vi "Replication and Deployment Utility.vi"() -> ()   [LabVIEW 2020]
uses:
  subVIs/Util/FP Control/FP Control Functions.ctl
  subVIs/rad_Globals.vi
  subVIs/Util/Controls/Exit Button.ctl
  <vilib>/Utility/miscctls.llb/LVRowAndColumnUnsignedTypeDef.ctl
  subVIs/Util/Controls/Refresh Button.ctl
  subVIs/Util/Controls/Retrieve Button.ctl
  subVIs/Util/Controls/Configure Button.ctl
  subVIs/TypeDefs/rad_State Data.ctl
  subVIs/App Images/TypeDefs/rad_Application Image Properties.ctl
  subVIs/App Images/TypeDefs/rad_App Images Settings.ctl
  subVIs/Targets/TypeDefs/rad_Targets Settings.ctl
  subVIs/App Images/TypeDefs/rad_AppImage Information.ctl
  subVIs/Util/Controls/Deploy Button.ctl
  subVIs/Util/Controls/Select All Button.ctl
  subVIs/App Images/TypeDefs/rad_FPGA Properties.ctl
  subVIs/App Images/TypeDefs/rad_FPGA Flash Properties.ctl
  subVIs/Util/Controls/Add Target Button.ctl
  subVIs/Targets/TypeDefs/rad_Target Information.ctl
  subVIs/Targets/TypeDefs/rad_Target Network Settings.ctl
panel:
  in  "Password":string
  in  "Targets Settings":bool
  in  "Refresh Targets":T1
  in  "Target List":i32[](listbox)
  in  "Add Target":T2
  in  "Select All":T3
  in  "Configure Targets":T4
  in  "Deploy":T5
  in  "Retrieve":T6
  in  "State":T7={"Targets Settings"={"Target Types"=["cRIO"], "Reduce Discovery Timeout"=TRUE}, "Targets Information"=[], "App Images Settings"={"App Images Folder"=path "C:/work/cRIO images", "App Images Temp Folder"=path "C:/Users/admin/AppData/Local/Temp/lvtemporary_671449.rad", "CurrentVersion"=""}, "App Images Information"=[], "Filtered Targets"=[], "AppMode"="Manager", "Configuration File Path"=path "C:/work/zaphiro_gtools/Sources/Utilities/rad_16_0_source/rad_config.ini", "Permissions"={"Retrieve AppImgs"=TRUE}, "User Added Targets"=["169.254.1.19"]} {"Targets Information"."Primary NIC"."IP Address Request Mode" items=["Static"=1, "DHCP/Link-Local"=2, "Link-Local Only"=4, "DHCP Only"=8]}
  in  "App Images Settings":bool
  in  "Refresh Apps":T1
  in  "Exit":T16
  in  "App Images List":i32(listbox)=-1
  in  "Configure App":T4
  # "Deployment Targets"
  # "Application Images"
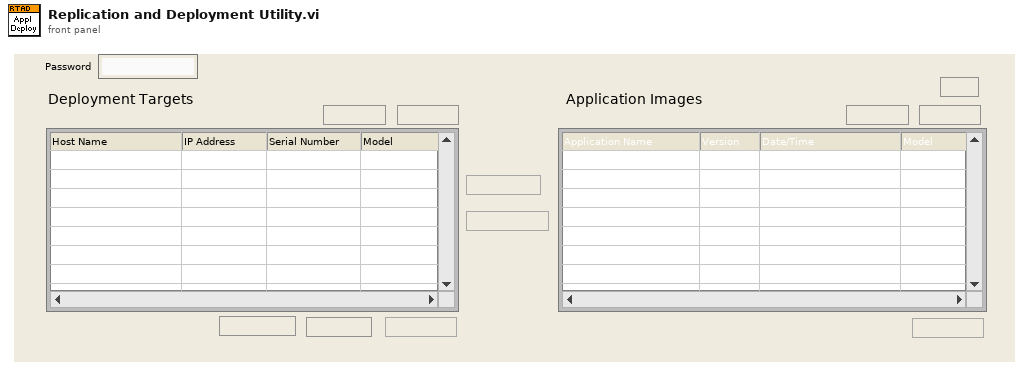
[diagram p1: front panel]
types:
  T1 = typedef "Refresh Button.ctl" = bool
  T2 = typedef "Add Target Button.ctl" = bool
  T3 = typedef "Select All Button.ctl" = bool
  T4 = typedef "Configure Button.ctl" = bool
  T5 = typedef "Deploy Button.ctl" = bool
  T6 = typedef "Retrieve Button.ctl" = bool
  T7 = typedef "rad_State Data.ctl" = cluster{"Targets Settings":T8, "Targets Information":T9[], "App Images Settings":T11, "App Images Information":T12[], "Filtered Targets":i32[], "AppMode":string, "Configuration File Path":path, "Permissions":cluster{"Retrieve AppImgs":bool}, "User Added Targets":string[]}
  T8 = typedef "rad_Targets Settings.ctl" = cluster{"Target Types":string[], "Reduce Discovery Timeout":bool}
  T9 = typedef "rad_Target Information.ctl" = cluster{"Hostname":string, "Serial number":string, "Product name":string, "Product code":i32, "System status":string, "Credential type":enum16{"None/Unlocked", "FTP Password", "NIAuth Credentials"}, "User added?":bool, "Primary NIC":T10}
  T10 = typedef "rad_Target Network Settings.ctl" = cluster{"MAC address":string, "IP Address Request Mode":i32, "IP address":string, "Subnet mask":string, "Gateway":string, "DNS server":string}
  T11 = typedef "rad_App Images Settings.ctl" = cluster{"App Images Folder":path, "App Images Temp Folder":path, "CurrentVersion":string}
  T12 = typedef "rad_AppImage Information.ctl" = cluster{"AppImage Properties":T13, "AppImage Path":path}
  T13 = typedef "rad_Application Image Properties.ctl" = cluster{"Name":string, "Version":string, "Time":timestamp, "Description":string, "Key":string, "Chassis":string, "FPGA Properties":T14, "Model":string, "Retrieve":string[], "Deploy":string[], "Installed Software":string[]}
  T14 = typedef "rad_FPGA Properties.ctl" = T15[]
  T15 = typedef "rad_FPGA Flash Properties.ctl" = cluster{"Resource Name":string, "Path":path}
  T16 = typedef "Exit Button.ctl" = bool
  T17 = typedef "LVPoint32TypeDef.ctl" = cluster{"Horizontal":i32, "Vertical":i32}
  T18 = typedef "LVRowAndColumnTypeDef.ctl" = cluster{"Row":i32, "Column":i32}
  T19 = typedef "FP Control Functions.ctl" = enum16{"Open", "Close", "Bring To Front", "Center"}
  T20 = typedef "LVRowAndColumnUnsignedTypeDef.ctl" = cluster{"Row":u32, "Column":u32}
  T21 = enum8{"Enabled", "Disabled", "Disabled and Grayed Out"}
  T22 = enum32{"invalid app kind", "Development System", "Run Time System", "Student Edition", "Embedded LabVIEW", "Evaluation", "Custom"}
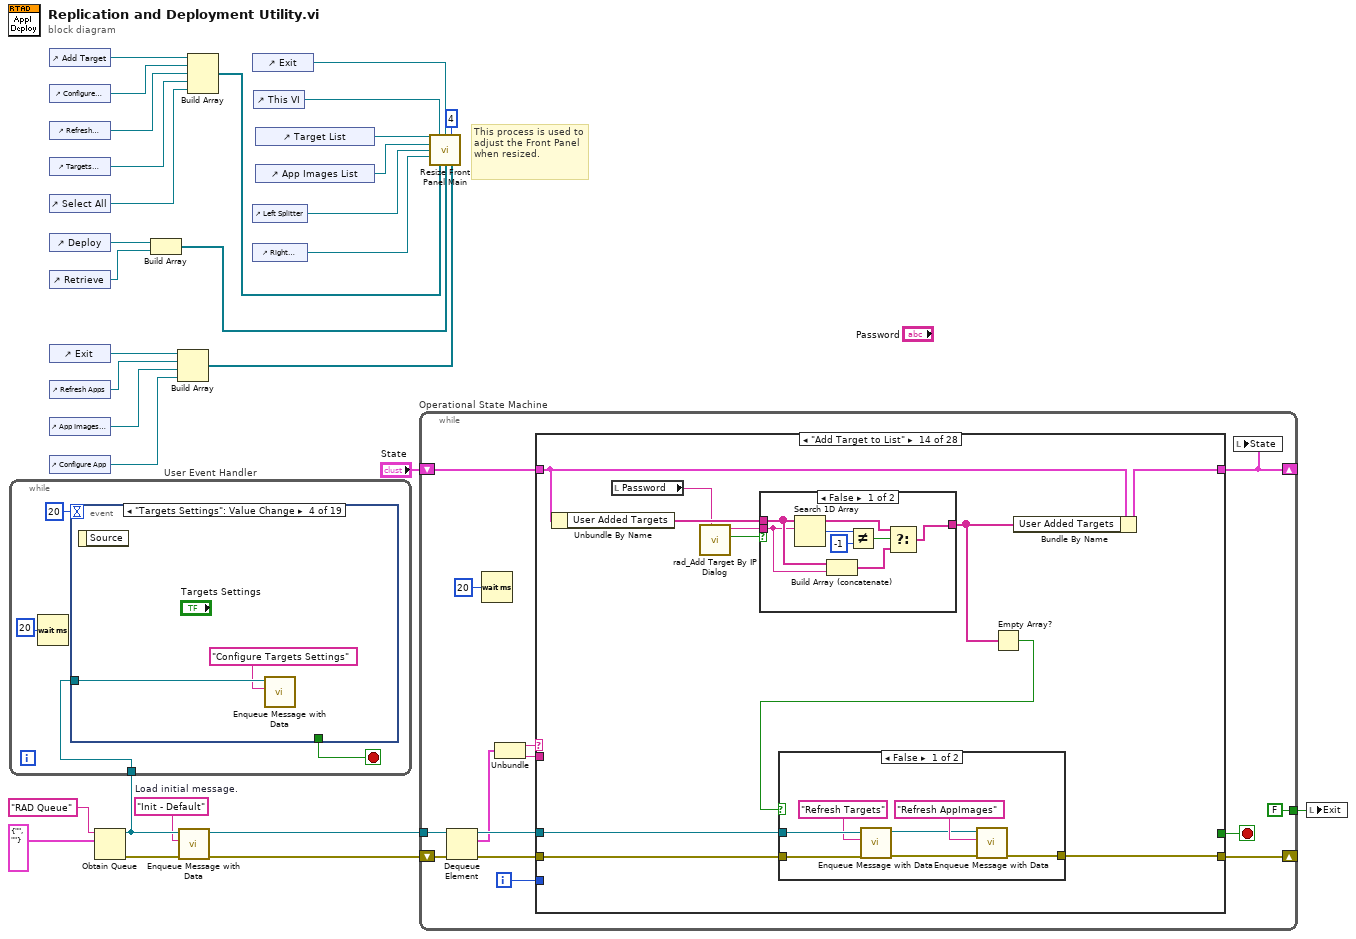
[diagram p0: block diagram]
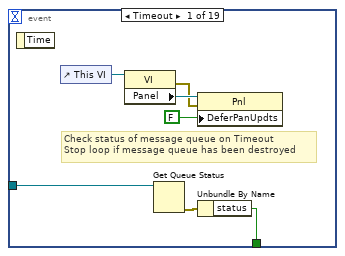
[diagram p2: hidden frame]
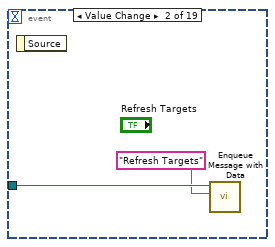
[diagram p3: hidden frame]
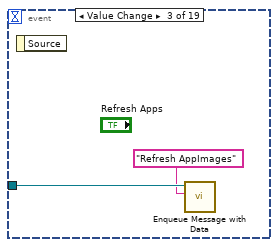
[diagram p4: hidden frame]
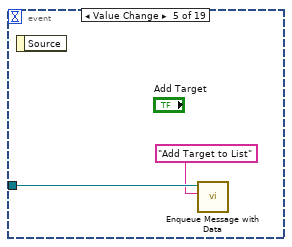
[diagram p5: hidden frame]
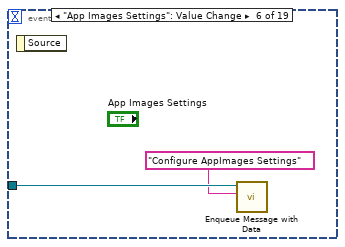
[diagram p6: hidden frame]
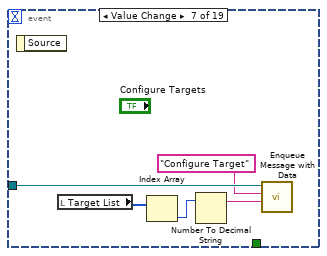
[diagram p7: hidden frame]
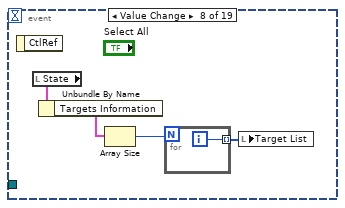
[diagram p8: hidden frame]
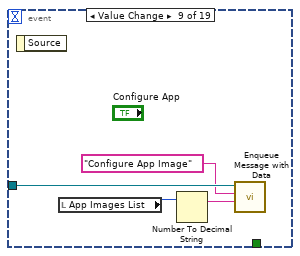
[diagram p9: hidden frame]
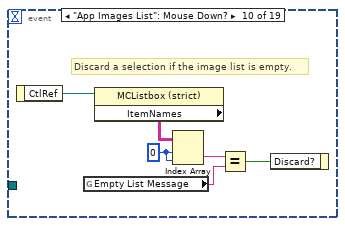
[diagram p10: hidden frame]
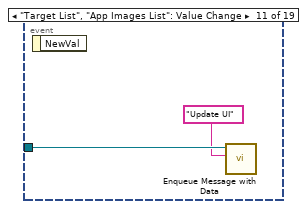
[diagram p11: hidden frame]
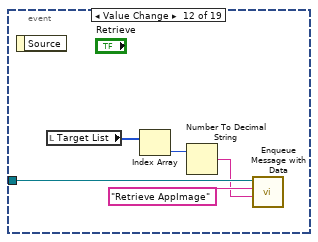
[diagram p12: hidden frame]
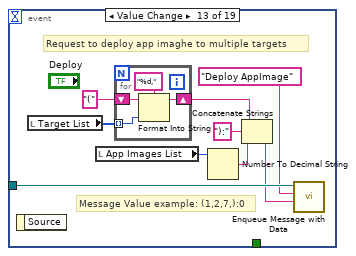
[diagram p13: hidden frame]
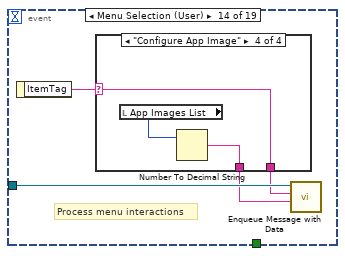
[diagram p14: hidden frame]
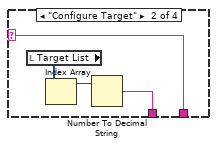
[diagram p16: hidden frame]
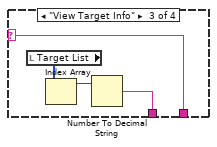
[diagram p17: hidden frame]
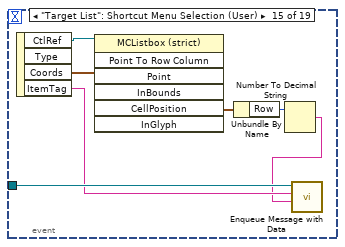
[diagram p18: hidden frame]
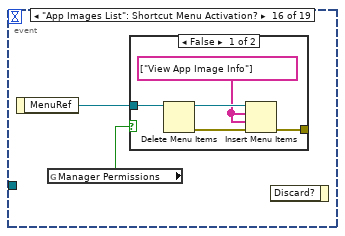
[diagram p19: hidden frame]
diagram:
  w3 = "Init - Default"  # Load initial message.
  # "This process is used to adjust the Front Panel when resized."
  n1 = control-ref of="Add Target"() -> (w21:refnum<vi>)
  n2 = control-ref of="Configure Targets"() -> (w20:refnum<vi>)
  n3 = control-ref of="Refresh Targets"() -> (w19:refnum<vi>)
  n4 = control-ref of="Targets Settings"() -> (w18:refnum<vi>)
  n5 = control-ref of="Select All"() -> (w17:refnum<vi>)
  n6 = control-ref of="Deploy"() -> (w15:refnum<vi>)
  n7 = control-ref of="Retrieve"() -> (w14:refnum<vi>)
  n8 = control-ref of="Exit"() -> (w12:refnum<vi>)
  n9 = control-ref of="Refresh Apps"() -> (w11:refnum<vi>)
  n10 = control-ref of="App Images Settings"() -> (w10:refnum<vi>)
  n11 = control-ref of="Configure App"() -> (w9:refnum<vi>)
  n12 = Obtain Queue(name (unnamed)="RAD Queue" ("message queue name"), element data type=cluster{string, string} {"", ""}) -> (queue out=w6:refnum<queue>, error out=w5:errorcluster)  [unwired: 3 in, 1 out]
  n13 = while "User Event Handler" {
    tunnel: w6 -> [w32]
    stop <- w33 stop-if-true
    n14 = Wait (ms)(milliseconds to wait=u32 20) -> ()  [unwired: 1 out]
    n15 = event shown="[3] \"Targets Settings\": Value Change" {
      selector: _ -> [_ _ _ _ _ _ _ _ _ _ _ _ _ _ _ _ _ _ _]
      dyn-events: _ -> [_ _ _ _ _ _ _ _ _ _ _ _ _ _ _ _ _ _ _]
      timeout: 20 -> [_ _ _ _ _ _ _ _ _ _ _ _ _ _ _ _ _ _ _]
      tunnel: [w39 _ _ _ _ _ _ _ _ _ _ _ _ _ _ _ _ TRUE ("Discard?") w139] -> w33
      tunnel: w32 -> [w41 w43 w45 w47 w49 w51 w54 _ w64 _ w73 w76 w81 w94 w110 _ w129 w135 w138]
      event Timeout {
        # "Check status of message queue on Timeout\nStop loop if message queue has been destroyed"
        n16 = event-data() -> ()  [unwired: 2 out]
        n17 = control-ref of="This VI"() -> (w35:refnum<vi>)
        n18 = property class="VI"(reference=w35) -> (error out=w36:errorcluster, "Panel"=w38:refnum<vi>)  [unwired: 1 in, 1 out]
        n19 = Get Queue Status(queue=w41) -> (error out=w40:errorcluster)  [unwired: 1 in, 8 out]
        n20 = property class="Pnl"(reference=w38, error in=w36, "DeferPanUpdts"=FALSE ("Defer Panel Updates")) -> ()  [unwired: 2 out]
        n21 = Unbundle By Name(w40) -> ("status"=w39:bool)
      }
      event Value Change {
        n22 = event-data() -> ()  [unwired: 2 out]
        n23 = call "Enqueue Message with Data.vi"("message ID"="Refresh Targets", "queue in"=w43) -> ()  [unwired: 8 in, 2 out]
      }
      event Value Change {
        n24 = event-data() -> ()  [unwired: 2 out]
        n25 = call "Enqueue Message with Data.vi"("message ID"="Refresh AppImages", "queue in"=w45) -> ()  [unwired: 8 in, 2 out]
      }
      event "Targets Settings": Value Change {
        n26 = event-data() -> ()  [unwired: 2 out]
        n27 = call "Enqueue Message with Data.vi"("message ID"="Configure Targets Settings", "queue in"=w47) -> ()  [unwired: 8 in, 2 out]
      }
      event Value Change {
        n28 = event-data() -> ()  [unwired: 2 out]
        n29 = call "Enqueue Message with Data.vi"("message ID"="Add Target to List" ("Message Name"), "queue in"=w49) -> ()  [unwired: 8 in, 2 out]
      }
      event "App Images Settings": Value Change {
        n30 = event-data() -> ()  [unwired: 2 out]
        n31 = call "Enqueue Message with Data.vi"("message ID"="Configure AppImages Settings", "queue in"=w51) -> ()  [unwired: 8 in, 2 out]
      }
      event Value Change {
        n32 = event-data() -> ()  [unwired: 2 out]
        n33 = local read "Target List"() -> (w55:i32[])
        n34 = Index Array(array=w55) -> (element=w56:i32)  [unwired: 1 in]
        n35 = Number To Decimal String(number=w56) -> (decimal integer string=w52:string)  [unwired: 1 out]
        n36 = call "Enqueue Message with Data.vi"("extra data"=w52, "message ID"="Configure Target", "queue in"=w54) -> ()  [unwired: 7 in, 2 out]
      }
      event Value Change {
        n37 = event-data() -> ()  [unwired: 2 out]
        n38 = local read "State"() -> (w59:T7)
        n39 = Unbundle By Name(w59) -> ("Targets Information"=w58:T9[])
        n40 = Array Size(array=w58) -> (size(s)=w57:i32)
        n41 = for {
          N: w57 -> [_]
          tunnel: [w61] -> w60 mode=indexing
          i -> [w61]
        }
        n42 = local write "Target List"(w60) -> ()
      }
      event Value Change {
        n43 = event-data() -> ()  [unwired: 2 out]
        n44 = local read "App Images List"() -> (w65:i32)
        n45 = Number To Decimal String(number=w65) -> (decimal integer string=w62:string)  [unwired: 1 out]
        n46 = call "Enqueue Message with Data.vi"("extra data"=w62, "message ID"="Configure App Image", "queue in"=w64) -> ()  [unwired: 7 in, 2 out]
      }
      event "App Images List": Mouse Down? {
        w69 = 0 ("index (row)")
        # "Discard a selection if the image list is empty."
        n47 = event-data() -> ("CtlRef"=w71:refnum<vi>)  [unwired: 1 out]
        n48 = global read "rad_Globals.vi" "Empty List Message"() -> (w67:string)
        n49 = property class="MCListbox (strict)"(reference=w71) -> ("ItemNames"=w70:string[][])  [unwired: 1 in, 2 out]
        n50 = Index Array(array=w70, index (row)=w69, index (col)=w69) -> (element=w68:string)
        n51 = Equal?(x=w68, y=w67) -> (x = y?=w66:bool)
        n52 = event-data("Discard?"=w66) -> ()  [unwired: 1 in, 1 out]
      }
      event "Target List", "App Images List": Value Change {
        n53 = event-data() -> ()  [unwired: 2 out]
        n54 = call "Enqueue Message with Data.vi"("message ID"="Update UI" ("Message"), "queue in"=w73) -> ()  [unwired: 8 in, 2 out]
      }
      event Value Change {
        n55 = event-data() -> ()  [unwired: 2 out]
        n56 = local read "Target List"() -> (w77:i32[])
        n57 = Index Array(array=w77) -> (element=w78:i32)  [unwired: 1 in]
        n58 = Number To Decimal String(number=w78) -> (decimal integer string=w74:string)  [unwired: 1 out]
        n59 = call "Enqueue Message with Data.vi"("extra data"=w74, "message ID"="Retrieve AppImage", "queue in"=w76) -> ()  [unwired: 7 in, 2 out]
      }
      event Value Change {
        # "Request to deploy app imaghe to multiple targets"
        # "Message Value example: (1,2,7,):0"
        n60 = event-data() -> ()  [unwired: 2 out]
        n61 = local read "Target List"() -> (w83:i32[])
        n62 = local read "App Images List"() -> (w85:i32)
        n63 = for {
          shift-right: [w91] -> w82
          shift-left: "(" -> [w89]
          tunnel: w83 -> [w90] mode=indexing
          n64 = Format Into String(format string="%d,", initial string=w89, w90) -> (resulting string=w91:string)  [unwired: 1 in, 1 out]
        }
        n65 = Number To Decimal String(number=w85) -> (decimal integer string=w86:string)  [unwired: 1 out]
        n66 = Concatenate Strings(w82, "):" ("string"), w86) -> (w79:string)
        n67 = call "Enqueue Message with Data.vi"("extra data"=w79, "message ID"="Deploy AppImage", "queue in"=w81) -> ()  [unwired: 7 in, 2 out]
      }
      event Menu Selection (User) {
        # "Process menu interactions"
        n68 = event-data() -> ("ItemTag"=w95:string)  [unwired: 1 out]
        n69 = case shown="\"Configure App Image\"" w95 {
          selector: w95 -> [w96 w98 w102 w106]
          tunnel: [w96 w98 w102 w106] -> w93
          tunnel: [_ w97 w101 w105] -> w92
          frame Default {
          }
          frame "Configure Target" {
            n70 = local read "Target List"() -> (w100:i32[])
            n71 = Index Array(array=w100) -> (element=w99:i32)  [unwired: 1 in]
            n72 = Number To Decimal String(number=w99) -> (decimal integer string=w97:string)  [unwired: 1 out]
          }
          frame "View Target Info" {
            n73 = local read "Target List"() -> (w104:i32[])
            n74 = Index Array(array=w104) -> (element=w103:i32)  [unwired: 1 in]
            n75 = Number To Decimal String(number=w103) -> (decimal integer string=w101:string)  [unwired: 1 out]
          }
          frame "Configure App Image" {
            n76 = local read "App Images List"() -> (w107:i32)
            n77 = Number To Decimal String(number=w107) -> (decimal integer string=w105:string)  [unwired: 1 out]
          }
        }
        n78 = call "Enqueue Message with Data.vi"("extra data"=w92, "message ID"=w93, "queue in"=w94) -> ()  [unwired: 7 in, 2 out]
      }
      event "Target List": Shortcut Menu Selection (User) {
        n79 = event-data() -> ("CtlRef"=w112:refnum<vi>, "Coords"=w111:T17, "ItemTag"=w109:string)  [unwired: 2 out]
        n80 = invoke class="MCListbox (strict)" method="Point To Row Column"(reference=w112, "Point"=w111) -> ("CellPosition"=w114:T18)  [unwired: 5 in, 6 out]
        n81 = Unbundle By Name(w114) -> ("Row"=w113:i32)
        n82 = Number To Decimal String(number=w113) -> (decimal integer string=w108:string)  [unwired: 1 out]
        n83 = call "Enqueue Message with Data.vi"("extra data"=w108, "message ID"=w109, "queue in"=w110) -> ()  [unwired: 7 in, 2 out]
      }
      event "App Images List": Shortcut Menu Activation? {
        n84 = event-data() -> ("MenuRef"=w116:refnum<k9>)  [unwired: 1 out]
        n85 = global read "rad_Globals.vi" "Manager Permissions"() -> (w115:bool)
        n86 = case shown="False" w115 {
          tunnel: w116 -> [w121 _]
          tunnel: [w118 _] -> _
          frame False {
            w117 = string[] ["View App Image Info"] ("item names")
            n87 = Delete Menu Items(9:w121) -> (0:w119:errorcluster, 3:w120:refnum<k9>)  [unwired: 3 in]
            n88 = Insert Menu Items(6:w119, 7:w117, 8:w117, 9:w120) -> (0:w118:errorcluster)  [unwired: 2 in, 2 out]
          }
          frame True {
          }
        }
        n89 = event-data() -> ()  [unwired: 2 in, 1 out]
      }
      event "App Images List": Shortcut Menu Selection (User) {
        n90 = event-data() -> ("CtlRef"=w131:refnum<vi>, "Coords"=w130:T17, "ItemTag"=w122:string)  [unwired: 1 out]
        n91 = Equal?(x=w122, y="Compare App Image") -> (x = y?=w127:bool)
        n92 = invoke class="MCListbox (strict)" method="Point To Row Column"(reference=w131, "Point"=w130) -> ("CellPosition"=w133:T18)  [unwired: 5 in, 6 out]
        n93 = Unbundle By Name(w133) -> ("Row"=w132:i32)
        n94 = Number To Decimal String(number=w132) -> (decimal integer string=w124:string)  [unwired: 1 out]
        n95 = Concatenate Strings("Only Image Selected(" ("string"), w124) -> (w126:string)
        n96 = Select(t=w126, s=w127, f=w124) -> (s? t:f=w123:string)
        n97 = call "Enqueue Message with Data.vi"("extra data"=w123, "message ID"=w122, "queue in"=w129) -> ()  [unwired: 7 in, 2 out]
      }
      event Value Change {
        n98 = event-data() -> ()  [unwired: 2 out]
        n99 = call "Enqueue Message with Data.vi"("message ID"="Exit", "queue in"=w135) -> ()  [unwired: 8 in, 2 out]
      }
      event Panel Close? {
        w139 = TRUE ("Discard?")
        # "Intercepts the upper right close panel\noperation to allow a smooth shutdown\nas opposed to immediately killing the app."
        n100 = event-data() -> ()  [unwired: 2 out]
        n101 = call "Enqueue Message with Data.vi"("message ID"="Exit", "queue in"=w138) -> ()  [unwired: 8 in, 2 out]
        n102 = event-data("Discard?"=w139) -> ()  [unwired: 1 in, 1 out]
      }
    }
  }
  n103 = Build Array(w15, w14) -> (w13:refnum<vi>[])
  n104 = Build Array(w12, w11, w10, w9) -> (w8:refnum<vi>[])
  n105 = call "Enqueue Message with Data.vi"("error in (no error)"=w5, "message ID"=w3, "queue in"=w6) -> ("error out"=w1:errorcluster, "queue out"=w2:refnum<queue>)  [unwired: 7 in]
  n106 = Build Array(w21, w20, w19, w18, w17) -> (w16:refnum<vi>[])
  n107 = control-ref of="Exit"() -> (w27:refnum<vi>)
  n108 = control-ref of="Left Splitter"() -> (w23:refnum<vi>)
  n109 = control-ref of="Right Splitter"() -> (w22:refnum<vi>)
  n110 = control-ref of="This VI"() -> (w26:refnum<vi>)
  n111 = control-ref of="Target List"() -> (w25:refnum<vi>)
  n112 = control-ref of="App Images List"() -> (w24:refnum<vi>)
  n113 = while "Operational State Machine" {
    shift-left: w1 -> [w145]
    shift-right: [w146] -> _
    tunnel: w2 -> [w150]
    shift-left: "State" -> [w153]
    shift-right: [w147] -> _
    tunnel: [T16 FALSE ("Exit")] -> w7
    i -> [w149]
    stop <- w143 stop-if-true
    n114 = Dequeue Element(queue=w150, error in (no error)=w145) -> (queue out=w152:refnum<queue>, element=w148:cluster{string, string}, error out=w151:errorcluster)  [unwired: 1 in, 1 out]
    n115 = Wait (ms)(milliseconds to wait=u32 20) -> ()  [unwired: 1 out]
    n116 = Unbundle(w148) -> (w142:string, w141:string)
    n117 = case shown="\"Add Target to List\"" w142 {
      tunnel: [w155 w157 w171 w181 w187 w208 w237 w252 w254 w258 w266 w278 w288 w305 w331 w347 w364 w377 w388 w390 w411 w426 w438 w456 w472 w502 w513 w520] -> w147
      tunnel: w153 -> [w155 w157 w175 w180 w188 w204 w237 w252 w254 w258 w266 w278 w289 w306 w332 w348 w364 w382 w388 w394 w412 w425 w438 w456 w473 w502 w513 w520]
      tunnel: w152 -> [_ _ w159 _ _ w200 _ _ _ _ w273 _ w286 w302 w330 w346 _ w376 _ w392 w405 w428 _ w443 w476 _ w514 _]
      tunnel: w151 -> [w154 w156 w164 w179 w186 w202 w234 w253 w255 w257 w272 w277 w285 w304 w326 w345 w357 w375 w387 w391 w407 w427 w439 w445 w479 w490 w518 w519]
      tunnel: w149 -> [_ _ _ _ _ _ _ _ _ _ _ _ _ _ _ _ _ _ _ _ _ _ _ _ _ _ _ _]
      tunnel: w141 -> [_ _ _ _ _ _ _ _ _ _ _ _ _ _ w340 _ w362 w386 _ _ w415 _ w435 w454 w481 w501 _ _]
      tunnel: [w154 w156 w158 w178 w186 w201 w220 w253 w255 errorcluster {"status"=FALSE, "code"=0, "source"=""} ("error out") w267 w277 w287 w303 w328 w342 w357 w374 w387 w393 w406 w422 w439 w444 w477 w489 w515 w519] -> w146
      tunnel: [_ _ _ _ _ _ _ _ _ _ TRUE _ _ _ _ _ _ _ _ _ _ _ _ _ _ _ _ _] -> w143
      frame "Missing Message Handler", Default {
      }
      frame "**** General Application Messages ****" {
      }
      frame "Init - Default" {
        w165 = T20 {"Row"=0, "Column"=0} ("Top Left Visible Cell")
        w167 = string[][] [] ("Item Names")
        w174 = u8 2 ("Disabled")
        # "Initialize the UI"
        # "Application Folder"
        # "Default AppImages folder"
        n118 = call "Util_App Application Directory.vi"() -> ("Application Directory"=w170:path)  [unwired: 11 out]
        n119 = call "Enqueue Message with Data.vi"("error in (no error)"=w164, "message ID"="Init - Load Config", "queue in"=w159) -> ("error out"=w163:errorcluster, "queue out"=w162:refnum<queue>)  [unwired: 7 in]
        n120 = local write "App Images List"(-1 ("App Images List")) -> ()
        n121 = local write "Target List"(i32[] [] ("Target List")) -> ()
        n122 = Build Path(base path=w170, name or relative path="appimages") -> (appended path=w176:path)
        n123 = Build Path(base path=w170, name or relative path="rad_config.ini" ("Config File Name")) -> (appended path=w168:path)
        n124 = call "Enqueue Message with Data.vi"("error in (no error)"=w163, "message ID"="Init - Configure Settings", "queue in"=w162) -> ("error out"=w158:errorcluster)  [unwired: 7 in, 1 out]
        n125 = property on="Configure App" class="Bool"("Disabled"=w174) -> ()  [unwired: 2 in, 2 out]
        n126 = property on="Configure Targets" class="Bool"("Disabled"=w174) -> ()  [unwired: 2 in, 2 out]
        n127 = Bundle By Name(cluster=w175, "App Images Settings.App Images Folder"=w176, "Configuration File Path"=w168) -> (w171:T7)
        n128 = property on="Target List" class="MCListbox (strict)"("ItemNames"=w167, "TopLeft"=w165) -> ()  [unwired: 2 in, 2 out]
        n129 = property on="App Images List" class="MCListbox (strict)"("ItemNames"=w167, "TopLeft"=w165) -> ()  [unwired: 2 in, 2 out]
        n130 = call "Util_FP Control.vi"("Function"=FP_Control_Functions."Center") -> ()  [unwired: 10 in, 1 out]
      }
      frame "Init - Load Config" {
        n131 = call "rad_Load Config.vi"("error in (no error"=w179, "State in"=w180) -> ("error out"=w178:errorcluster, "State out"=w181:T7)  [unwired: 1 in, 7 out]
      }
      frame "Init - Configure Settings" {
        # "The temp folder should always be writable."
        # "Set permissions and update UI based on application\nmode. Disable or hide controls not appropriate\nfor current application mode."
        # "Apply configuration settings from config file"
        n132 = Unbundle By Name(w188) -> ("AppMode"=w189:string)
        n133 = case shown="\"Manager\"" w189 {
          tunnel: [TRUE ("Visible") FALSE ("Visible")] -> w185
          frame "Manager" {
          }
          frame Default {
          }
        }
        n134 = call <vilib>:"Generate Temporary File Path.vi"("Temporary File Extension (tmp)"="rad") -> ("Unique Temporary File Path"=w182:path)  [unwired: 9 in, 1 out]
        n135 = property on="Retrieve" class="Bool"("Visible"=w185) -> ()  [unwired: 2 in, 2 out]
        n136 = property on="Configure App" class="Bool"("Visible"=w185) -> ()  [unwired: 2 in, 2 out]
        n137 = global write "rad_Globals.vi" "Manager Permissions"(w185) -> ()
        n138 = global write "rad_Globals.vi" "ShownImageVersionDialog"(FALSE ("ShownNewerVersionDialog")) -> ()
        n139 = Bundle By Name(cluster=w188, "App Images Settings.App Images Temp Folder"=w182, "Permissions.Retrieve AppImgs"=w185) -> (w187:T7)
      }
      frame "Update UI" {
        # "Scroll the lists to the top if no item is selected."
        # "Display target and app images based on settings\nfor each of these tables"
        n140 = Unbundle By Name(w204) -> ("Targets Information"=w211:T9[], "Targets Settings.Target Types"=w203:string[], "App Images Information"=w205:T12[])
        n141 = call "rad_Format Application Images Information.vi"("App Images Information"=w205) -> ("App Images Information"=w206:string[][])  [unwired: 10 out]
        n142 = call "rad_FilterTargets.vi"("Target Types"=w203, "Targets Information"=w211) -> ("Filtered Targets"=w209:i32[], "Targets Information"=w210:T9[])  [unwired: 8 out]
        n143 = Bundle By Name(cluster=w204, "Filtered Targets"=w209) -> (w208:T7)
        n144 = call "rad_Format Target Information.vi"("Targets Information"=w210) -> ("Targets Information"=w207:string[][])  [unwired: 10 out]
        n145 = property on="App Images List" class="MCListbox (strict)"("ItemNames"=w206) -> (error out=w197:errorcluster)  [unwired: 2 in, 1 out]
        n146 = property on="Target List" class="MCListbox (strict)"("ItemNames"=w207) -> (error out=w198:errorcluster)  [unwired: 2 in, 1 out]
        n147 = flat-sequence {
          tunnel: w198 -> [_]
          tunnel: w197 -> [_]
          tunnel: ["App Images List"] -> w195
          tunnel: [w215] -> w196
          tunnel: [-1 ("y")] -> w193
          frame #0 {
            n148 = Array Size(array="Target List") -> (size(s)=w215:i32)
          }
        }
        n149 = Equal?(x=w195, y=w193) -> (x = y?=w192:bool)
        n150 = Equal To 0?(x=w196) -> (x = 0?=w194:bool)
        n151 = call "Enqueue Message with Data.vi"("error in (no error)"=w202, "message ID"="Update Buttons and Menus" ("Message Name"), "queue in"=w200) -> ("error out"=w201:errorcluster)  [unwired: 7 in, 1 out]
        n152 = case shown="True" w192 {
          frame False {
          }
          frame True {
            n153 = property on="App Images List" class="MCListbox (strict)"("TopLeft"=T20 {"Row"=0, "Column"=0} ("Top Left Visible Cell")) -> ()  [unwired: 2 in, 2 out]
          }
        }
        n154 = case shown="True" w194 {
          frame False {
          }
          frame True {
            n155 = property on="Target List" class="MCListbox (strict)"("TopLeft"=T20 {"Row"=0, "Column"=0} ("Top Left Visible Cell")) -> ()  [unwired: 2 in, 2 out]
          }
        }
      }
      frame "Update Buttons and Menus" {
        w223 = T21."Disabled and Grayed Out" ("Disabled")
        w224 = T21."Enabled" ("Disabled")
        # "Enable and disable buttons and \nenu items based on selections\nin both tables"
        n156 = local read "App Images List"() -> (w235:i32)
        n157 = local read "Target List"() -> (w236:i32[])
        n158 = Unbundle By Name(w237) -> ("Permissions.Retrieve AppImgs"=w218:bool)
        n159 = call "rad_Button and Menu Status.vi"("Manager Permissions"=w218, "App Image List"=w235, "Target List"=w236) -> ("Retrieve AppImage"=w226:bool, "Deploy AppImage"=w228:bool, "View Target Info"=w233:bool, "Configure App Image"=w230:bool, "Configure Target"=w232:bool)  [unwired: 3 in, 1 out]
        n160 = Current VI's Menubar() -> (w238:refnum<k9>)
        n161 = Set Menu Item Info(7:"Configure Target" ("item tag"), 8:w234, 9:w232, 11:w238) -> (0:w240:errorcluster, 3:w242:refnum<k9>)  [unwired: 3 out]
        n162 = Select(t=w224, s=w232, f=w223) -> (s? t:f=w231:T21)
        n163 = Select(t=w224, s=w230, f=w223) -> (s? t:f=w229:T21)
        n164 = Select(t=w224, s=w228, f=w223) -> (s? t:f=w227:T21)
        n165 = Select(t=w224, s=w226, f=w223) -> (s? t:f=w225:T21)
        n166 = Set Menu Item Info(7:"Configure App Image" ("item tag"), 8:w240, 9:w230, 11:w242) -> (0:w243:errorcluster, 3:w244:refnum<k9>)  [unwired: 3 out]
        n167 = Set Menu Item Info(7:"View Target Info" ("item tag"), 8:w243, 9:w233, 11:w244) -> (0:w245:errorcluster, 3:w246:refnum<k9>)  [unwired: 3 out]
        n168 = Set Menu Item Info(7:"Deploy AppImage" ("item tag"), 8:w245, 9:w228, 11:w246) -> (0:w247:errorcluster, 3:w248:refnum<k9>)  [unwired: 3 out]
        n169 = property on="Configure Targets" class="Bool"("Disabled"=w231) -> ()  [unwired: 2 in, 2 out]
        n170 = property on="Configure App" class="Bool"("Disabled"=w229) -> ()  [unwired: 2 in, 2 out]
        n171 = property on="Deploy" class="Bool"("Disabled"=w227) -> ()  [unwired: 2 in, 2 out]
        n172 = property on="Retrieve" class="Bool"("Disabled"=w225) -> ()  [unwired: 2 in, 2 out]
        n173 = Set Menu Item Info(7:"Retrieve AppImage" ("item tag"), 8:w247, 9:w226, 11:w248) -> (0:w221:errorcluster, 3:w222:refnum<k9>)  [unwired: 3 out]
        n174 = Set Menu Item Info(7:"Convert Images" ("item tag"), 8:w221, 9:w218, 11:w222) -> (0:w220:errorcluster)  [unwired: 4 out]
      }
      frame "Status" {
      }
      frame "About" {
        # "Show About dialog"
        n175 = call "rad_About Dialog.vi"() -> ()  [unwired: 12 out]
      }
      frame "Error" {
        # "Display run-time error message\nAdd code to log error if desired"
        n176 = disable-structure shown="TARGET_TYPE==Windows" {
          disable-tunnel: w257 -> [w259 _]
          frame condition #0 (active) {
            n177 = call <vilib>:"Simple Error Handler.vi"("error in (no error)"=w259) -> ()  [unwired: 1 in, 8 out]
          }
          frame condition #1 {
          }
        }
      }
      frame "Exit" {
        w260 = T20 {"Row"=0, "Column"=0} ("Top Left Visible Cell")
        w261 = string[][] [] ("Item Names")
        # "Store current settings in the application config file"
        # "Close the front panel if the application is running as an EXE"
        n178 = Release Queue(queue=w273, force destroy? (F)=TRUE, error in (no error)=w272) -> (error out=w265:errorcluster)  [unwired: 2 out]
        n179 = Open Application Reference() -> (0:w270:errorcluster, 3:w271:refnum<vi>)  [unwired: 4 in]
        n180 = call "rad_Save Config.vi"("error in (no error"=w265, "State"=w266) -> ("error out"=w264:errorcluster)  [unwired: 1 in, 8 out]
        n181 = property class="App"(reference=w271, error in=w270) -> ("App.Kind"=w269:T22)  [unwired: 2 out]
        n182 = case shown="\"Run Time System\"" w269 {
          frame Default {
          }
          frame "Run Time System" {
            # "Close FP in EXE"
            n183 = Current VI's Path() -> (path=w276:path)
            n184 = Open VI Reference(vi path=w276) -> (vi reference=w275:refnum<vi>, error out=w274:errorcluster)  [unwired: 5 in]
            n185 = invoke class="VI" method="FP.Close"(reference=w275, error in=w274) -> ()  [unwired: 1 in, 3 out]
          }
        }
        n186 = property on="Exit" class="Bool (strict)"(error in=w264, "Val(Sgnl)"=TRUE) -> (error out=w267:errorcluster)  [unwired: 1 in, 1 out]
        n187 = property on="Target List" class="MCListbox (strict)"("ItemNames"=w261, "TopLeft"=w260) -> ()  [unwired: 2 in, 2 out]
        n188 = property on="App Images List" class="MCListbox (strict)"("ItemNames"=w261, "TopLeft"=w260) -> ()  [unwired: 2 in, 2 out]
      }
      frame "**** Target Messages ****" {
      }
      frame "Refresh Targets" {
        # "Refresh list of RT targets on the local subnet.\nShow progress dialog during this process."
        n189 = Unbundle By Name(w289) -> ("Targets Settings.Reduce Discovery Timeout"=w282:bool, "User Added Targets"=w294:string[], "Targets Settings.Target Types"=w281:string[])
        n190 = local read "Password"() -> (w279:string)
        n191 = call "Util_Progress Show Progress Popup.vi"("error in (no error)"=w285, "Title"="Discovering Targets", "Message"="Refreshing target list...") -> ("error out"=w283:errorcluster)  [unwired: 1 in, 7 out]
        n192 = Search 1D Array(1D array=w281, element="User Targets Only") -> (index of element=w291:i32)  [unwired: 1 in]
        n193 = Not Equal?(x=w291, y=-1) -> ()  [unwired: 1 out]
        n194 = call "rad_Refresh Target Information.vi"("Password"=w279, "Reduce Discovery Timeout"=w282, "error in (no error)"=w283, "User Added Targets Only"=TRUE, "User Added Targets"=w294) -> ("error out"=w284:errorcluster, "Targets Information"=w293:T9[])  [unwired: 5 in]
        n195 = call "Util_Progress Close Progress Popup.vi"("error in (no error)"=w284) -> ()  [unwired: 2 in, 9 out]
        n196 = Bundle By Name(cluster=w289, "Targets Information"=w293) -> (w288:T7)
        n197 = call "Enqueue Message with Data.vi"("error in (no error)"=w284, "message ID"="Update UI", "queue in"=w286) -> ("error out"=w287:errorcluster)  [unwired: 7 in, 1 out]
      }
      frame "Add Target to List" {
        n198 = Unbundle By Name(w306) -> ("User Added Targets"=w308:string[])
        n199 = local read "Password"() -> (w298:string)
        n200 = call "rad_Add Target By IP Dialog.vi"("Password"=w298) -> ("Canceled?"=w301:bool, "IP Address"=w307:string)  [unwired: 9 in]
        n201 = case shown="False" w301 {
          tunnel: w308 -> [w319 w324]
          tunnel: w307 -> [w318 _]
          tunnel: [w320 w324] -> w300
          frame False {
            n202 = Search 1D Array(1D array=w319, element=w318) -> (index of element=w323:i32)  [unwired: 1 in]
            n203 = Build Array (concatenate)(w319, w318) -> (w317:string[])
            n204 = Not Equal?(x=w323, y=-1) -> (x != y?=w321:bool)
            n205 = Select(t=w319, s=w321, f=w317) -> (s? t:f=w320:string[])
          }
          frame True {
          }
        }
        n206 = Empty Array?(array=w300) -> (empty?=w299:bool)
        n207 = case shown="False" w299 {
          tunnel: w304 -> [w315 w316]
          tunnel: [w309 w316] -> w303
          tunnel: w302 -> [w314 _]
          frame False {
            n208 = call "Enqueue Message with Data.vi"("error in (no error)"=w315, "message ID"="Refresh Targets" ("Message Name"), "queue in"=w314) -> ("error out"=w311:errorcluster, "queue out"=w310:refnum<queue>)  [unwired: 7 in]
            n209 = call "Enqueue Message with Data.vi"("error in (no error)"=w311, "message ID"="Refresh AppImages" ("Message Name"), "queue in"=w310) -> ("error out"=w309:errorcluster)  [unwired: 7 in, 1 out]
          }
          frame True {
          }
        }
        n210 = Bundle By Name(cluster=w306, "User Added Targets"=w300) -> (w305:T7)
      }
      frame "Configure Target" {
        # "Update network settings/configuration of the selected RT target"
        n211 = Unbundle By Name(w332) -> ("Targets Information"=w336:T9[], "Filtered Targets"=w339:i32[])
        n212 = Decimal String To Number(string=w340) -> (number=w338:i32)  [unwired: 3 out]
        n213 = local read "Password"() -> (w325:string)
        n214 = Index Array(array=w339, index=w338) -> (element=w334:i32)
        n215 = Index Array(array=w336, index=w334) -> (element=w337:T9)
        n216 = call "rad_Configure Target Dialog.vi"("Password"=w325, "Error In"=w326, "Target Information in"=w337) -> ("Error Out"=w327:errorcluster, "Target Information out"=w335:T9)  [unwired: 7 out]
        n217 = Replace Array Subset(array=w336, new element=w335, index=w334) -> (w333:T9[])
        n218 = call <vilib>:"General Error Handler.vi"("error in (no error)"=w327) -> ()  [unwired: 10 in, 5 out]
        n219 = Bundle By Name(cluster=w332, "Targets Information"=w333) -> (w331:T7)
        n220 = call "Enqueue Message with Data.vi"("error in (no error)"=w326, "message ID"="Update UI", "queue in"=w330) -> ("error out"=w328:errorcluster)  [unwired: 7 in, 1 out]
      }
      frame "Configure Targets Settings" {
        # "Update the RT Target settings >> select which types of RT targets to display in the table\nCompactRIO, PXI, FieldPoint, or Other"
        n221 = Unbundle By Name(w348) -> ("Targets Settings"=w343:T8)
        n222 = call "rad_Configure Targets Settings Dialog.vi"("Targets Settings"=w343) -> ("Targets Settings"=w344:T8)  [unwired: 10 out]
        n223 = Equal?(x=w344, y=w343) -> (x = y?=w341:bool)
        n224 = Bundle By Name(cluster=w348, "Targets Settings"=w344) -> (w347:T7)
        n225 = case shown="False" w341 {
          tunnel: w346 -> [w352 _]
          tunnel: w345 -> [w351 w353]
          tunnel: [w350 w353] -> w342
          frame False {
            n226 = call "Enqueue Message with Data.vi"("error in (no error)"=w351, "message ID"="Update UI", "queue in"=w352) -> ("error out"=w350:errorcluster)  [unwired: 7 in, 1 out]
          }
          frame True {
          }
        }
      }
      frame "View Target Info" {
        # "Display additional information about the selected RT target in a popup window"
        n227 = Unbundle By Name(w364) -> ("Targets Information"=w363:T9[], "Filtered Targets"=w361:i32[])
        n228 = Decimal String To Number(string=w362) -> (number=w360:i32)  [unwired: 3 out]
        n229 = Index Array(array=w361, index=w360) -> (element=w359:i32)
        n230 = Index Array(array=w363, index=w359) -> (element=w355:T9)
        n231 = local read "Password"() -> (w354:string)
        n232 = call "rad_Get Target Info (IP).vi"("Password"=w354, "error in (no error)"=w357, "Target settings in"=w355) -> ("error out"=w356:errorcluster, "Target settings out"=w358:T9)  [unwired: 7 in]
        n233 = case shown="No Error" w356 {
          selector: w356 -> [_ w366]
          tunnel: w358 -> [w365 _]
          frame No Error {
            n234 = call "rad_Target Info Dialog.vi"("Target Information"=w365) -> ()  [unwired: 11 out]
          }
          frame Error {
            n235 = call <vilib>:"General Error Handler.vi"("error in (no error)"=w366) -> ()  [unwired: 10 in, 5 out]
          }
        }
      }
      frame "Delete Target" {
        n236 = Unbundle By Name(w382) -> ("Targets Information"=w381:T9[], "Filtered Targets"=w369:i32[], "User Added Targets"=w370:string[])
        n237 = Decimal String To Number(string=w386) -> (number=w372:i32)  [unwired: 2 in, 1 out]
        n238 = Index Array(array=w369, index=w372) -> (element=w371:i32)
        n239 = Delete From Array(array=w381, length=1, index=w371) -> (deleted portion=w379:T9[], array with subset deleted=w380:T9[])
        n240 = Index Array(array=w379) -> (element=w378:T9)  [unwired: 1 in]
        n241 = Unbundle By Name(w378) -> ("Primary NIC.IP address"=w368:string)
        n242 = Search 1D Array(1D array=w370, element=w368) -> (index of element=w385:i32)  [unwired: 1 in]
        n243 = call "Enqueue Message with Data.vi"("error in (no error)"=w375, "message ID"="Update UI" ("Message Name"), "queue in"=w376) -> ("error out"=w374:errorcluster)  [unwired: 7 in, 1 out]
        n244 = Delete From Array(array=w370, length=1, index=w385) -> (array with subset deleted=w367:string[])  [unwired: 1 out]
        n245 = Bundle By Name(cluster=w382, "Targets Information"=w380, "User Added Targets"=w367) -> (w377:T7)
      }
      frame "**** Image Messages ****" {
      }
      frame "Refresh AppImages" {
        # "Update list of application images available in the configured folder"
        n246 = Unbundle By Name(w394) -> ("App Images Settings.App Images Temp Folder"=w395:path, "App Images Settings.App Images Folder"=w399:path)
        n247 = call "Util_Progress Show Progress Popup.vi"("Title"="Refreshing App Images", "Message"="Refreshing application images list...") -> ("error out"=w398:errorcluster)  [unwired: 2 in, 7 out]
        n248 = call "rad_List Application Images.vi"("App Image Temp Folder"=w395, "error in (no error)"=w398, "App Images Folder"=w399) -> ("error out"=w397:errorcluster, "Application Images Infomration"=w396:T12[])  [unwired: 1 in, 6 out]
        n249 = Bundle By Name(cluster=w394, "App Images Information"=w396) -> (w390:T7)
        n250 = call "Util_Progress Close Progress Popup.vi"("error in (no error)"=w397) -> ()  [unwired: 2 in, 9 out]
        n251 = call "Enqueue Message with Data.vi"("error in (no error)"=w391, "message ID"="Update UI" ("Message"), "queue in"=w392) -> ("error out"=w393:errorcluster)  [unwired: 7 in, 1 out]
      }
      frame "Configure App Image" {
        # "Update additional information (name, verison, description)\nstored with the selected application image"
        n252 = Unbundle By Name(w412) -> ("App Images Settings.App Images Temp Folder"=w408:path, "App Images Information"=w414:T12[])
        n253 = Decimal String To Number(string=w415) -> (number=w410:i32)  [unwired: 3 out]
        n254 = Index Array(array=w414, index=w410) -> (element=w409:T12)
        n255 = call "rad_Configure Application Image.vi"("Temp Folder"=w408, "error in (no error)"=w407, "App Images Information"=w409) -> ("error out"=w404:errorcluster, "Cancelled"=w402:bool, "App Images Information"=w403:T12)  [unwired: 6 in]
        n256 = Replace Array Subset(array=w414, new element=w403, index=w410) -> (w413:T12[])
        n257 = case shown="False" w402 {
          tunnel: [w419 w420] -> w406
          tunnel: w405 -> [w417 _]
          tunnel: w404 -> [w416 w420]
          frame False {
            n258 = call "Enqueue Message with Data.vi"("error in (no error)"=w416, "message ID"="Refresh AppImages", "queue in"=w417) -> ("error out"=w419:errorcluster)  [unwired: 7 in, 1 out]
          }
          frame True {
          }
        }
        n259 = Bundle By Name(cluster=w412, "App Images Information"=w413) -> (w411:T7)
      }
      frame "Configure AppImages Settings" {
        # "Update the selection of the folder where application images are stored"
        n260 = Unbundle By Name(w425) -> ("App Images Settings"=w424:T11)
        n261 = call "rad_Configure App Images Settings Dialog.vi"("App Images Settings"=w424) -> ("Cancelled"=w421:bool, "App Images Settings"=w423:T11)  [unwired: 1 in, 8 out]
        n262 = case shown="False" w421 {
          tunnel: w428 -> [w432 _]
          tunnel: w427 -> [w430 w433]
          tunnel: [w429 w433] -> w422
          frame False {
            n263 = call "Enqueue Message with Data.vi"("error in (no error)"=w430, "message ID"="Refresh AppImages", "queue in"=w432) -> ("error out"=w429:errorcluster)  [unwired: 7 in, 1 out]
          }
          frame True {
          }
        }
        n264 = Bundle By Name(cluster=w425, "App Images Settings"=w423) -> (w426:T7)
      }
      frame "View App Image Info" {
        n265 = Unbundle By Name(w438) -> ("App Images Information"=w437:T12[])
        n266 = Decimal String To Number(string=w435) -> (number=w434:i32)  [unwired: 2 in, 1 out]
        n267 = Index Array(array=w437, index=w434) -> (element=w436:T12)
        n268 = call "rad_View App Image Info.vi"("App Images Information"=w436) -> ()  [unwired: 11 in]
      }
      frame "Delete App Image" {
        n269 = Unbundle By Name(w456) -> ("App Images Information"=w455:T12[])
        n270 = Decimal String To Number(string=w454) -> (number=w453:i32)  [unwired: 2 in, 1 out]
        n271 = Index Array(array=w455, index=w453) -> (element=w452:T12)
        n272 = Unbundle By Name(w452) -> ("AppImage Path"=w447:path, "AppImage Properties.Name"=w449:string, "AppImage Properties.Version"=w440:string)
        n273 = Concatenate Strings("Are you sure you want to delete " ("string"), w449, " version " ("string"), w440, "?" ("string")) -> (w448:string)
        n274 = Two Button Dialog(message=w448, 2:"Delete" ("button name (\"OK\")")) -> (T button?=w446:bool)  [unwired: 1 in]
        n275 = case shown="True" w446 {
          tunnel: w447 -> [_ w463]
          tunnel: w445 -> [w457 w462]
          tunnel: [w457 w460] -> w444
          tunnel: w443 -> [_ w459]
          frame False {
          }
          frame True {
            n276 = Delete(path (use dialog)=w463, error in=w462) -> (error out=w461:errorcluster)  [unwired: 3 in, 2 out]
            n277 = call "Enqueue Message with Data.vi"("error in (no error)"=w461, "message ID"="Refresh AppImages" ("Message Name"), "queue in"=w459) -> ("error out"=w460:errorcluster)  [unwired: 7 in, 1 out]
          }
        }
      }
      frame "Retrieve AppImage" {
        # "Retrieve the application image\nfrom the selected RT target."
        n278 = Unbundle By Name(w473) -> ("App Images Settings.App Images Temp Folder"=w475:path, "App Images Settings.App Images Folder"=w469:path, "Targets Information"=w465:T9[], "Filtered Targets"=w466:i32[])
        n279 = Decimal String To Number(string=w481) -> (number=w480:i32)  [unwired: 3 out]
        n280 = local read "Password"() -> (w464:string)
        n281 = Index Array(array=w466, index=w480) -> (element=w482:i32)
        n282 = Index Array(array=w465, index=w482) -> (element=w467:T9)
        n283 = call "rad_Retrieve Application Image From Target.vi"("password"=w464, "App Images Temp Folder"=w475, "error in (no error)"=w479, "Target settings"=w467, "App Images Folder"=w469) -> ("error out"=w478:errorcluster, "Cancelled"=w470:bool, "New App Image Path"=w474:path)  [unwired: 2 in, 2 out]
        n284 = Strip Path(path=w474) -> (stripped path=w471:path)  [unwired: 1 out]
        n285 = case shown="True" w470 {
          tunnel: w478 -> [w486 w487]
          tunnel: [w485 w487] -> w477
          tunnel: w476 -> [w484 _]
          frame False {
            n286 = call "Enqueue Message with Data.vi"("error in (no error)"=w486, "message ID"="Refresh AppImages" ("Message Name"), "queue in"=w484) -> ("error out"=w485:errorcluster)  [unwired: 7 in, 1 out]
          }
          frame True {
          }
        }
        n287 = Select(t=w469, s=w470, f=w471) -> (s? t:f=w468:path)
        n288 = Bundle By Name(cluster=w473, "App Images Settings.App Images Folder"=w468) -> (w472:T7)
      }
      frame "Deploy AppImage" {
        # "Deploy the selected application image to the select RT target(s)"
        n289 = Unbundle By Name(w502) -> ("App Images Settings.App Images Temp Folder"=w492:path, "App Images Information"=w498:T12[], "Targets Information"=w494:T9[], "Filtered Targets"=w495:i32[])
        n290 = Scan From String(format string="(%[^)]):%d", input string=w501) -> (output 1=w497:string, output 2=w499:i32)  [unwired: 2 in, 5 out]
        n291 = while {
          shift-right: [w509] -> _
          shift-left: w497 -> [w511]
          tunnel: w495 -> [w506]
          tunnel: w494 -> [w504]
          tunnel: [w503] -> w491 mode=indexing
          stop <- w508 stop-if-true
          n292 = Scan From String(format string="%d,", input string=w511) -> (remaining string=w509:string, output 1=w505:i32)  [unwired: 2 in, 3 out]
          n293 = Index Array(array=w506, index=w505) -> (element=w507:i32)
          n294 = Empty String/Path?(string/path=w509) -> (empty?=w508:bool)
          n295 = Index Array(array=w504, index=w507) -> (element=w503:T9)
        }
        n296 = local read "Password"() -> (w488:string)
        n297 = Index Array(array=w498, index=w499) -> (element=w496:T12)
        n298 = Unbundle By Name(w496) -> ("AppImage Path"=w493:path)
        n299 = call "rad_Deploy Application Image.vi"("Password"=w488, "App Image Temp Folder"=w492, "error in (no error)"=w490, "Selected Targets"=w491, "App Image Path"=w493) -> ("error out"=w489:errorcluster)  [unwired: 6 out]
      }
      frame "Convert Images" {
        n300 = Unbundle By Name(w513) -> ("App Images Settings.App Images Folder"=w512:path)
        n301 = call "Util_ConvertImageToLatest.vi"("error in (no error)"=w518, "Image Path"=w512) -> ("error out"=w516:errorcluster)  [unwired: 9 in]
        n302 = call "Enqueue Message with Data.vi"("error in (no error)"=w516, "message ID"="Refresh AppImages" ("Message Name"), "queue in"=w514) -> ("error out"=w515:errorcluster)  [unwired: 7 in, 1 out]
      }
      frame "****Licence****" {
      }
    }
    n303 = local write "State"(w147) -> ()
  }
  n304 = call "Resize Front Panel Main.vi"("Left Listbox"=w25, "Top Level VI"=w26, "Stop"=w27, "Number of Columns"=4, "Right Listbox"=w24, "Left Splitter"=w23, "Right Splitter"=w22, "Left Pane Items"=w16, "Mid Pane Items"=w13, "Right Pane Items"=w8) -> ()  [unwired: 5 in, 1 out]
  n305 = local write "Exit"(w7) -> ()
